vi "CAN Read.vi"(8 "error in":errorcluster, 9 "TimestampBuffer":T1, 10 "MessageBuffer":T2, 11 "Channel":u16) -> (0 "error out":errorcluster, 1 "TimestampBuffer out":T1, 2 "MessageBuffer out":T2, 3 "function return":u32, 5 "Channel out":u16)   [LabVIEW 2023, in "PCAN2023.lvlib"]
doc: "Reads a CAN message from the receive queue of a PCAN Channel\n\n\nTPCANStatus __stdcall CAN_Read(\n TPCANHandle Channel, \n TPCANMsg* MessageBuffer, \n TPCANTimestamp* TimestampBuffer);"
uses:
  PCAN2023.lvlib
  PCANBasic.dll
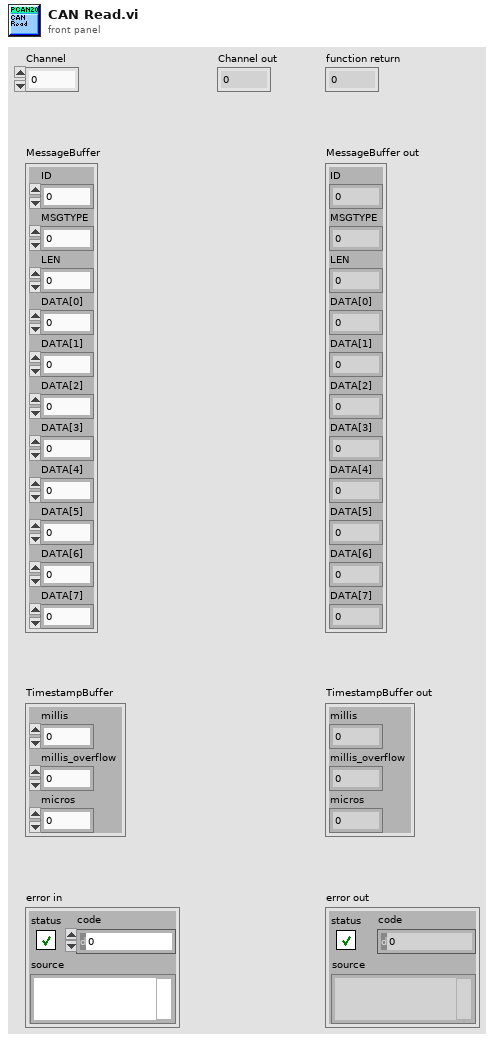
[diagram p1: front panel]
types:
  T1 = cluster{"millis":u32, "millis_overflow":u16, "micros":u16}
  T2 = cluster{"ID":u32, "MSGTYPE":u8, "LEN":u8, "DATA[0]":u8, "DATA[1]":u8, "DATA[2]":u8, "DATA[3]":u8, "DATA[4]":u8, "DATA[5]":u8, "DATA[6]":u8, "DATA[7]":u8}
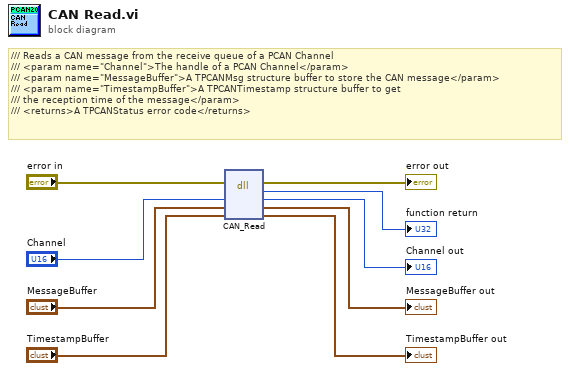
[diagram p0: block diagram]
diagram:
  # "/// Reads a CAN message from the receive queue of a PCAN Channel\n/// <param name=\"Channel\">The handle of a PCAN Channel</param>\n/// <param name=\"MessageBuffer\">A TPCANMsg structure buffer to store the CAN message</param>\n/// <param name=\"TimestampBuffer\">A TPCANTimestamp structure buffer to get\n/// the reception time of the message</param>\n/// <returns>A TPCANStatus error code</returns>"
  n1 = dll-call lib="D:/PEAK/PCAN2023/PCAN2023/PCANBasic.*" fn="CAN_Read"(error in="error in", "Channel"="Channel", "MessageBuffer"="MessageBuffer", "TimestampBuffer"="TimestampBuffer") -> (error out=→"error out":errorcluster, →"function return":u32, "Channel"=→"Channel out":u16, "MessageBuffer"=→"MessageBuffer out":T2, "TimestampBuffer"=→"TimestampBuffer out":T1)  [unwired: 2 in, 1 out]
